vi "Calculate-3D miniscan coordinate at Zplane intersection.vi"(5 "Abs. index of selected Z-plane (unity-based)":i32, 7 "Number of Z-planes":i32, 9 "Relative index of selected Z-plane (unity-based)":i32, 10 "Number of intersected Zplanes":i32, 11 "input cluster":T1 {"ROI group ID" format="%#_6f"; "Laser Power (%)" format="%#_6f"; "Zoom" format="%#_6f"; "Frame Size" format="%#_6f"; "Number of lines" format="%#_6f"; "Composite ID" format="%#_6f"; "Angle (deg)" format="%#_6f"; "ROI Time (ns)" format="%#_6f"; "ROI ID" format="%#_6f"; "Pixels in ROI" format="%#_6f"; "ROI index" format="%#_6f"; "Z stop" format="%#_6f"; "Y stop" format="%#_6f"; "X stop" format="%#_6f"; "Z start" format="%#_6f"; "X start" format="%#_6f"; "Y start" format="%#_6f"}) -> (3 "£D miniscan Z-plane intersection coordinates":cluster{"X":i32, "Y":i32})   [LabVIEW 2013]
uses:
  Typedefs/ROI parameters data type.ctl
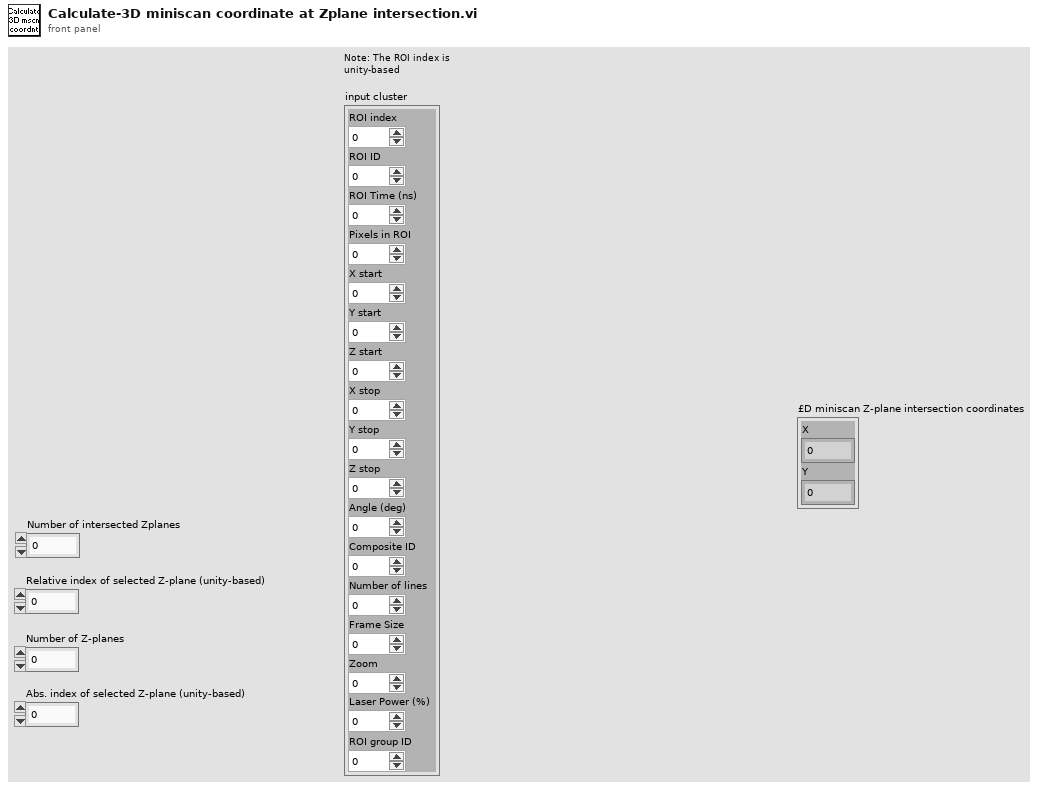
[diagram p1: front panel]
types:
  T1 = typedef "ROI parameters data type.ctl" = cluster{"ROI index":dbl, "ROI ID":dbl, "ROI Time (ns)":dbl, "Pixels in ROI":dbl, "X start":dbl, "Y start":dbl, "Z start":dbl, "X stop":dbl, "Y stop":dbl, "Z stop":dbl, "Angle (deg)":dbl, "Composite ID":dbl, "Number of lines":dbl, "Frame Size":dbl, "Zoom":dbl, "Laser Power (%)":dbl, "ROI group ID":dbl}
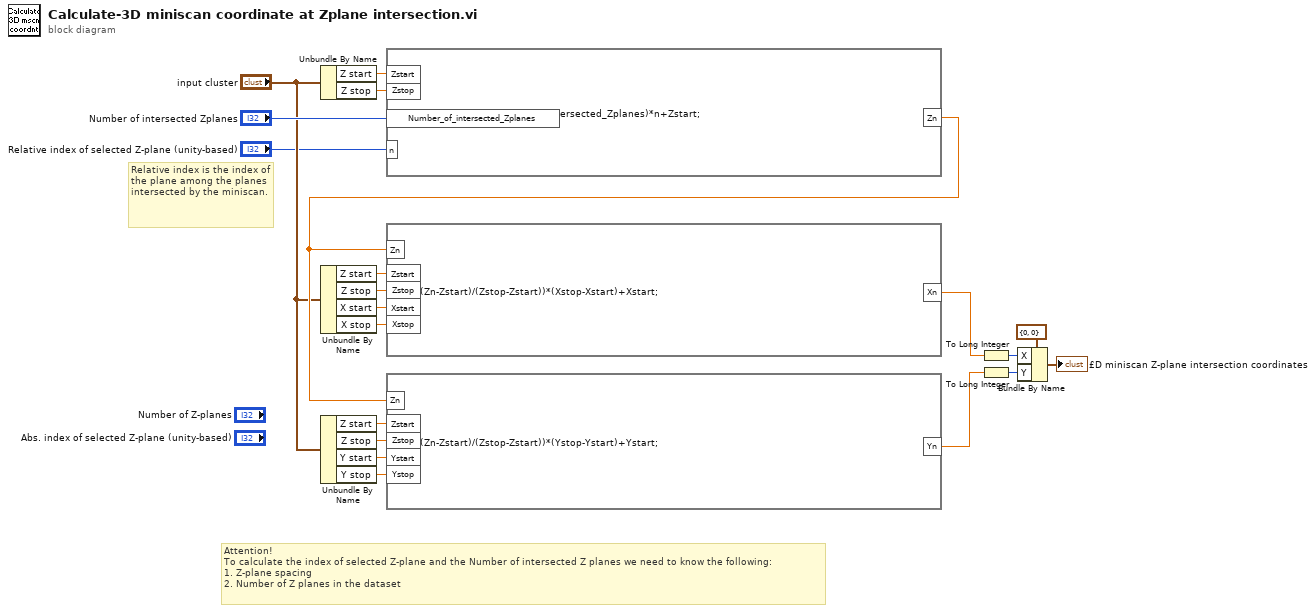
[diagram p0: block diagram]
diagram:
  # "Relative index is the index of the plane among the planes intersected by the miniscan."
  # "Attention!\nTo calculate the index of selected Z-plane and the Number of intersected Z planes we need to know the following:\n1. Z-plane spacing\n2. Number of Z planes in the dataset"
  n1 = Unbundle By Name("input cluster") -> ("Z start"=w16:dbl, "Z stop"=w15:dbl)
  n2 = Unbundle By Name("input cluster") -> ("Z start"=w10:dbl, "Z stop"=w11:dbl, "X start"=w9:dbl, "X stop"=w8:dbl)
  n3 = Unbundle By Name("input cluster") -> ("Z start"=w6:dbl, "Z stop"=w5:dbl, "Y start"=w3:dbl, "Y stop"=w4:dbl)
  n4 = formula code="Zn=((Zstop-Zstart)/Number_of_intersected_Zplanes)*n+Zstart;"("Zstop"=w15, "Zstart"=w16, "Number_of_intersected_Zplanes"="Number of intersected Zplanes", "n"="Relative index of selected Z-plane (unity-based)") -> ("Zn"=w7:dbl)
  n5 = formula code="Xn=((Zn-Zstart)/(Zstop-Zstart))*(Xstop-Xstart)+Xstart;"("Zstart"=w10, "Zn"=w7, "Zstop"=w11, "Xstart"=w9, "Xstop"=w8) -> ("Xn"=w13:dbl)
  n6 = formula code="Yn=((Zn-Zstart)/(Zstop-Zstart))*(Ystop-Ystart)+Ystart;"("Zstop"=w5, "Zstart"=w6, "Zn"=w7, "Ystart"=w3, "Ystop"=w4) -> ("Yn"=w12:dbl)
  n7 = To Long Integer(number=w13) -> (32bit integer=w17:i32)
  n8 = To Long Integer(number=w12) -> (32bit integer=w18:i32)
  n9 = Bundle By Name(cluster=cluster{"X":i32, "Y":i32} {"X"=0, "Y"=0} ("Point"), "X"=w17, "Y"=w18) -> (→"£D miniscan Z-plane intersection coordinates":cluster{"X":i32, "Y":i32})
